vi "dvp Vi Get Frame Count.vi"(10 "pFrameCount":T1, 11 "handle":u32) -> (2 "pFrameCount out":T1, 3 "function return":u32(ring))   [LabVIEW 2018, in "LabViewDVPCamera.lvlib"]
doc: "LabviewDvp2Api dvpStatus dvpViGetFrameCount(dvpHandle handle, dvpViFrameCount *pFrameCount);"
uses:
  LabViewDVPCamera.lvlib
  LabViewDVPCamera/LabViewDVPCamera.dll
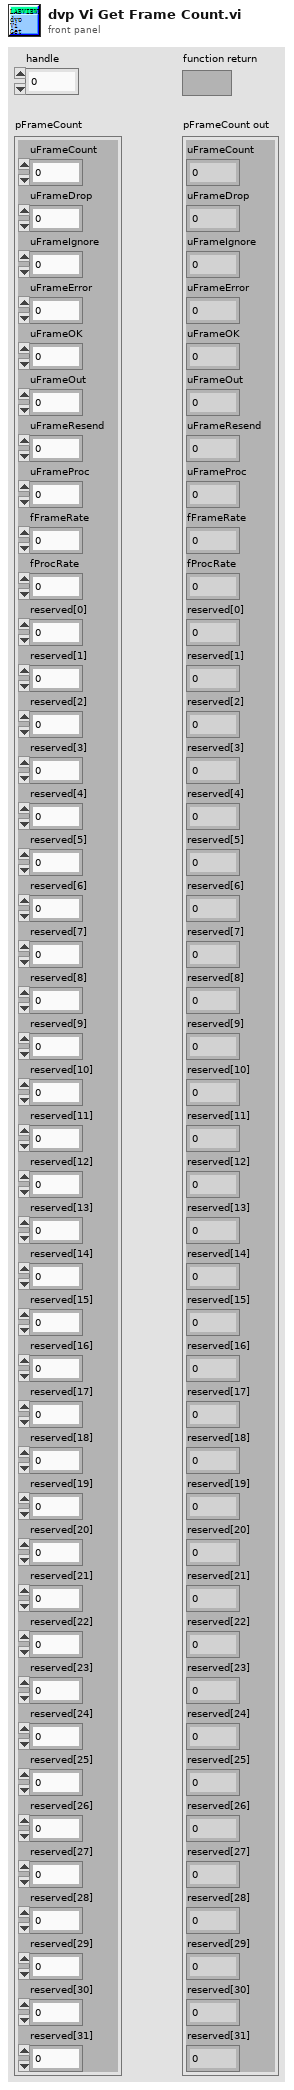
[diagram p1: front panel]
types:
  T1 = cluster{"uFrameCount":u32, "uFrameDrop":u32, "uFrameIgnore":u32, "uFrameError":u32, "uFrameOK":u32, "uFrameOut":u32, "uFrameResend":u32, "uFrameProc":u32, "fFrameRate":sgl, "fProcRate":sgl, "reserved[0]":i32, "reserved[1]":i32, "reserved[2]":i32, "reserved[3]":i32, "reserved[4]":i32, "reserved[5]":i32, "reserved[6]":i32, "reserved[7]":i32, "reserved[8]":i32, "reserved[9]":i32, "reserved[10]":i32, "reserved[11]":i32, "reserved[12]":i32, "reserved[13]":i32, "reserved[14]":i32, "reserved[15]":i32, "reserved[16]":i32, "reserved[17]":i32, "reserved[18]":i32, "reserved[19]":i32, "reserved[20]":i32, "reserved[21]":i32, "reserved[22]":i32, "reserved[23]":i32, "reserved[24]":i32, "reserved[25]":i32, "reserved[26]":i32, "reserved[27]":i32, "reserved[28]":i32, "reserved[29]":i32, "reserved[30]":i32, "reserved[31]":i32}
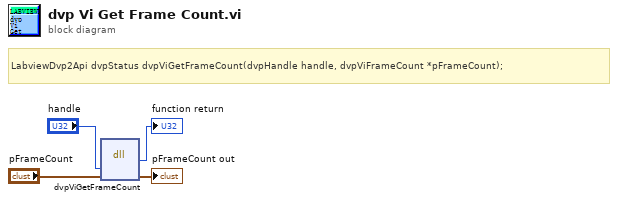
[diagram p0: block diagram]
diagram:
  # "LabviewDvp2Api dvpStatus dvpViGetFrameCount(dvpHandle handle, dvpViFrameCount *pFrameCount);"
  n1 = dll-call lib="C:/Program Files (x86)/DVP2 Labview cn 64/Sample/LabViewDVPCamera/LabViewDVPCamera.*" fn="dvpViGetFrameCount"("handle"="handle", "pFrameCount"="pFrameCount") -> (→"function return":u32, "pFrameCount"=→"pFrameCount out":T1)  [unwired: 4 in, 2 out]
